vi "Cache LLP Packet Word.vi"(0 "state in":T1={"llp packet cache"=[], "llp packet cache size"=0.0, "timestamp"={"valid"=FALSE, "count"=0.0, "id"=enum."SI0 LLP", "metadata"=0}, "packet bytes remaining"=0.0, "state"=enum."deserialize payload"}, 5 "llp packet word":u8[](array[numeric]), 9 "llp packet word valid":bool) -> (4 "state out":T1={"llp packet cache"=[], "llp packet cache size"=0.0, "timestamp"={"valid"=FALSE, "count"=0.0, "id"=enum."SI0 LLP", "metadata"=0}, "packet bytes remaining"=0.0, "state"=enum."deserialize payload"})   [LabVIEW 2020, in "GettingStarted_Common_148X_FPGA.lvlib"]
uses:
  <instrlib>/FlexRIO/CSI-2/v2/FPGA/Types/Deserialize LLP Packet State Data.ctl
  <instrlib>/FlexRIO/CSI-2/v2/FPGA/Types/FPGA LLP Packet Timestamp.ctl
  <instrlib>/FlexRIO/CSI-2/v2/FPGA/Types/Timestamp ID.ctl
  <instrlib>/FlexRIO/CSI-2/v2/FPGA/Types/Deserialize LLP Packet State.ctl
  GettingStarted_Common_148X_FPGA.lvlib
  <instrlib>/FlexRIO/CSI-2/v2/FPGA/NI CSI-2 API FPGA v2.lvlib
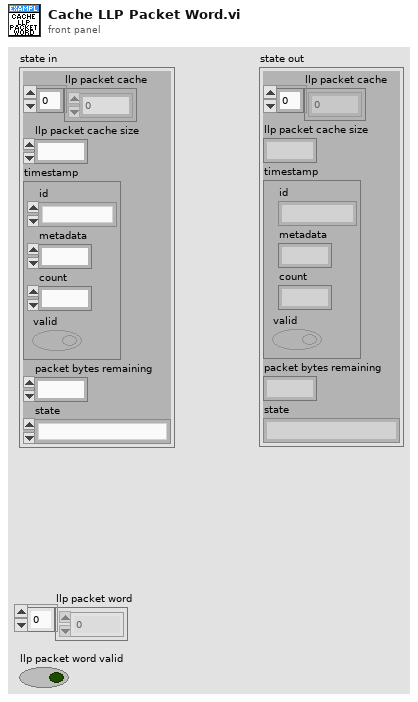
[diagram p1: front panel]
types:
  T1 = typedef "NI CSI-2 API FPGA v2.lvlib/Deserialize LLP Packet State Data.ctl" = cluster{"llp packet cache":u8[], "llp packet cache size":fxp<+,4,4>, "timestamp":T2, "packet bytes remaining":fxp<+,17,17>, "state":T4}
  T2 = typedef "NI CSI-2 API FPGA v2.lvlib/FPGA LLP Packet Timestamp.ctl" = cluster{"valid":bool, "count":fxp<+,50,50>, "id":T3, "metadata":u8}
  T3 = typedef "NI CSI-2 API FPGA v2.lvlib/Timestamp ID.ctl" = enum8{"SI0 LLP", "SI1 LLP", "SI2 LLP", "SI3 LLP", "SI4 LLP", "SI5 LLP", "SI6 LLP", "SI7 LLP", "SO0 LLP", "SO1 LLP", "SO2 LLP", "SO3 LLP", "SO4 LLP", "SO5 LLP", "SO6 LLP", "SO7 LLP", "Ser0 GPIO Bank", "Ser1 GPIO Bank", "Ser2 GPIO Bank", "Ser3 GPIO Bank", "Ser4 GPIO Bank", "Ser5 GPIO Bank", "Ser6 GPIO Bank", "Ser7 GPIO Bank", "Des0 GPIO Bank", "Des1 GPIO Bank", "Des2 GPIO Bank", "Des3 GPIO Bank", "Des4 GPIO Bank", "Des5 GPIO Bank", "Des6 GPIO Bank", "Des7 GPIO Bank", "User0", "User1", "User2", "User3", "User4", "User5", "User6", "User7", "User8", "User9", "User10", "User11", "User12", "User13", "User14", "User15", "User16", "User17", "User18", "User19", "User20", "User21", "User22", "User23", "User24", "User25", "User26", "User27", "User28", "User29", "User30", "User31"}
  T4 = typedef "NI CSI-2 API FPGA v2.lvlib/Deserialize LLP Packet State.ctl" = enum8{"deserialize timestamp", "deserialize size and header", "deserialize payload"}
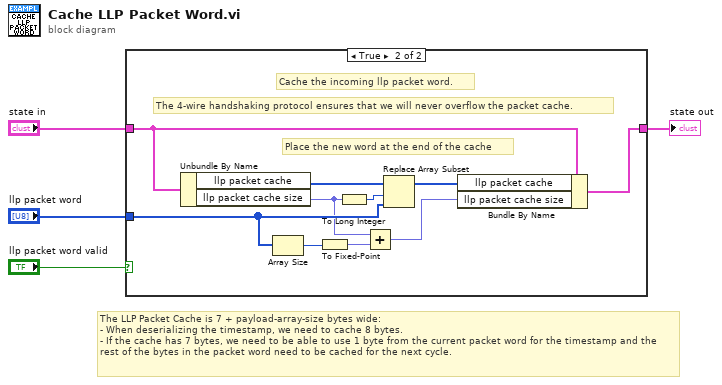
[diagram p0: block diagram]
diagram:
  # "The LLP Packet Cache is 7 + payload-array-size bytes wide:\n- When deserializing the timestamp, we need to cache 8 bytes.\n- If the cache has 7 bytes, we need to be able to use 1 byte from the current packet word for the timestamp and the rest of the bytes in the packet word need to be cached for the next cycle."
  n1 = case shown="True" "llp packet word valid" {
    tunnel: "llp packet word" -> [_ w15]
    tunnel: "state in" -> [w5 w14]
    tunnel: [w5 w13] -> w4
    frame False {
    }
    frame True {
      # "Place the new word at the end of the cache"
      # "Cache the incoming llp packet word."
      # "The 4-wire handshaking protocol ensures that we will never overflow the packet cache."
      n2 = Unbundle By Name(w14) -> ("llp packet cache"=w12:u8[], "llp packet cache size"=w10:fxp<+,4,4>)
      n3 = Array Size(array=w15) -> (size(s)=w7:i32)
      n4 = To Fixed-Point(number=w7) -> (fixed-point=w6:fxp<+,4,4>)  [unwired: 1 in]
      n5 = To Long Integer(number=w10) -> (32bit integer=w11:i32)
      n6 = Add(x=w10, y=w6) -> (x+y=w8:fxp<+,4,4>)
      n7 = Replace Array Subset(array=w12, new element=w15, index=w11) -> (w9:u8[])
      n8 = Bundle By Name(cluster=w14, "llp packet cache"=w9, "llp packet cache size"=w8) -> (w13:T1)
    }
  }
  "state out" <- w4
